vi "CFTS-Open Help Topic.vi"(7 "Topic Keyword":string) -> (15 "error out":errorcluster)   [LabVIEW 2020]
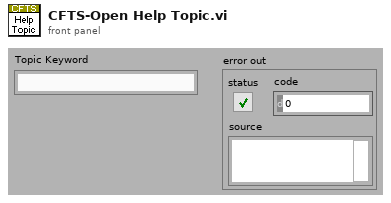
[diagram p1: front panel]
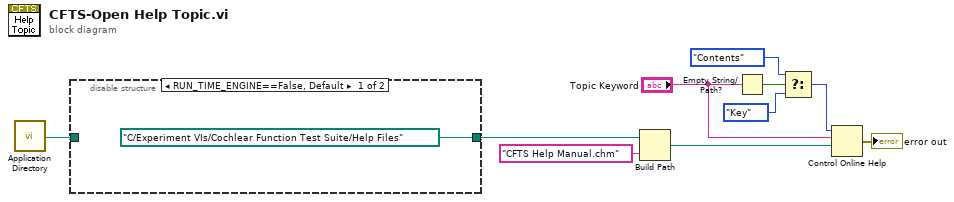
[diagram p0: block diagram]
diagram:
  n1 = call <vilib>:"Application Directory.vi"() -> ("Application Directory"=w8:path)
  n2 = disable-structure shown="RUN_TIME_ENGINE==False, Default" {
    disable-tunnel: [path "C:/Experiment VIs/Cochlear Function Test Suite/Help Files" ("acrobat document") w12] -> w9
    disable-tunnel: w8 -> [_ w12]
    frame condition #0 (active) {
    }
    frame condition #1 {
    }
  }
  n3 = Build Path(base path=w9, name or relative path="CFTS Help Manual.chm") -> (appended path=w7:path)
  n4 = Empty String/Path?(string/path="Topic Keyword") -> (empty?=w5:bool)
  n5 = Select(t=enum16{"Contents", "Key", "Close"}."Contents" ("Operation"), s=w5, f=enum16{"Contents", "Key", "Close"}."Key") -> (s? t:f=w3:enum16{"Contents", "Key", "Close"})
  n6 = Control Online Help(2:w7, 3:"Topic Keyword", 4:w3) -> (0:→"error out":errorcluster)  [unwired: 1 in]
